vi "CLSUIP_ResizeBDWin.vi"(7 "OverrideRetooler in":refnum<class "OverrideRetooler.lvclass">, 8 "error in (no error)":errorcluster, 11 "VI Refnum":refnum<vi>) -> (0 "error out":errorcluster, 3 "VI Refnum out":refnum<vi>)   [LabVIEW 2021, in "MemberVICreation.lvlib" / "OverrideRetooler.lvclass"]
uses:
  <resource>/Framework/Providers/LVClassLibrary/NewAccessors/OverrideRetooler/OverrideRetooler.lvclass
  <resource>/Framework/Providers/LVClassLibrary/NewAccessors/VIRetooler/VIRetooler.lvclass
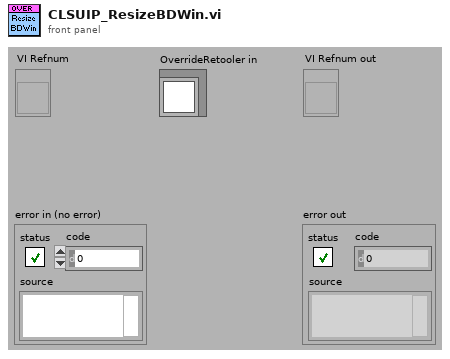
[diagram p1: front panel]
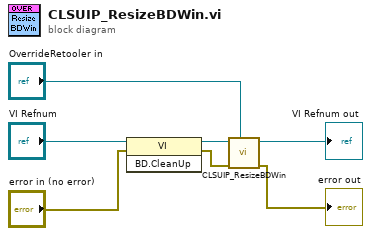
[diagram p0: block diagram]
diagram:
  n1 = invoke class="VI" method="BD.CleanUp"(reference="VI Refnum", error in="error in (no error)") -> (reference out=w1:refnum<vi>, error out=w2:errorcluster)  [unwired: 1 in, 1 out]
  n2 = call-parent "CLSUIP_ResizeBDWin.vi"("VIRetooler in"="OverrideRetooler in", "error in (no error)"=w2, "VI Refnum"=w1) -> ("error out"=→"error out":errorcluster, "VI Refnum out"=→"VI Refnum out":refnum<vi>)  [unwired: 7 out]
